vi "Koordinatenberechnung_Lichtgitter.vi"(8 "Fehler in":errorcluster, 11 "Cluster in":T1={"Initialisierung"={"Online?"=FALSE, "Grundpfad"=path "", "Kamera Oben"="", "IP-Adresse Flüssiglinse"="", "Flüssiglinse"=refnum, "Kamera Unten"="", "IP-Adresse SPS"="", "SPS-Verbindung"={"TCP Connection Ref"=refnum, "IP address"="", "timeout ms"=5000, "Connected?"=FALSE, "PLC Type"=enum."S7 1200", "Rack S7 400"=0, "Slot S7 400"=0, "PDU Size"=0, "connection semaphore"=refnum}, "IP-Adresse Lichtgitter"="", "Lichtgitter"=refnum, "Skalierungsfaktor"=0.0, "Bilder Oben"=[], "Bild Unten"=refnum, "Bild Ausschnitt Unten"=refnum}, "Einstellungen"={"Gesamtablauf gestartet"=FALSE, "i. O. Bilder speichern"=FALSE, "Bildspeicherung Offline"=FALSE, "Ausgewähltes Offline-Datum"="", "Ausgewähltes Offline-Teil"="", "Speicherpfad Bilder"=path ""}, "Artikeldaten"={"Artikelnummer"="", "Fertigungsauftrag"="", "Muster ISO"=refnum, "Belichtungszeit Referenzmarken"=0.0, "Fokus Referenzmarken"=0.0, "Belichtungszeit ISO"=0.0, "Fokus ISO"=0.0, "Belichtungszeit Unten"=0.0, "Kontaktanzahl"=0, "Aktueller Kontakt"=0, "Kontaktposition"={"x"=0.0, "y"=0.0}, "Winkel ISO"=0.0, "ISO-Muster nicht vorhanden"=FALSE}, "Werte Kamera Oben"={"Koordinatensystem"={"Punkt x-Achse"={"X"=0.0, "Y"=0.0}, "Ursprung"={"X"=0.0, "Y"=0.0}, "Punkt y-Achse"={"X"=0.0, "Y"=0.0}}, "Position Kontakt"={"x"=0.0, "y"=0.0}, "Winkel Kontakt"=0.0}, "Werte Kamera Unten"={"Prüfung Unten n. i. O."=FALSE}, "Werte Lichtgitter"={"Messwerte Referenzmarken"=[], "Mittelpunkt Referenzmarken"={"x"=0.0, "y"=0.0}, "Messwerte Kontakt"=[], "Offset"={"x"=0.0, "y"=0.0}}, "Rückmeldungen"={"Koordinaten ermittelt"=FALSE, "Vermessung Lichtgitter fertig"=FALSE, "Nachkontrolle Kamera Unten fertig"=FALSE}, "Fehler"={"Referenzen nicht gefunden"=FALSE, "Kontakt nicht gefunden"=FALSE, "Referenzen nicht in Lichtgitter"=FALSE, "Kontakt zu groß"=FALSE, "Kontakt zu klein"=FALSE}, "Statistik"={"Statistiken"=[]}, "Timer"={"Timer Start Position"=0, "Timer Start Lichtgitter"=0, "Timer Start Kamera Unten"=0}}) -> (0 "Fehler out":errorcluster, 2 "Durchmesser Kontakt (mm)":dbl format="%#.3g", 3 "Cluster out":T1={"Initialisierung"={"Online?"=FALSE, "Grundpfad"=path "", "Kamera Oben"="", "IP-Adresse Flüssiglinse"="", "Flüssiglinse"=refnum, "Kamera Unten"="", "IP-Adresse SPS"="", "SPS-Verbindung"={"TCP Connection Ref"=refnum, "IP address"="", "timeout ms"=5000, "Connected?"=FALSE, "PLC Type"=enum."S7 1200", "Rack S7 400"=0, "Slot S7 400"=0, "PDU Size"=0, "connection semaphore"=refnum}, "IP-Adresse Lichtgitter"="", "Lichtgitter"=refnum, "Skalierungsfaktor"=0.0, "Bilder Oben"=[], "Bild Unten"=refnum, "Bild Ausschnitt Unten"=refnum}, "Einstellungen"={"Gesamtablauf gestartet"=FALSE, "i. O. Bilder speichern"=FALSE, "Bildspeicherung Offline"=FALSE, "Ausgewähltes Offline-Datum"="", "Ausgewähltes Offline-Teil"="", "Speicherpfad Bilder"=path ""}, "Artikeldaten"={"Artikelnummer"="", "Fertigungsauftrag"="", "Muster ISO"=refnum, "Belichtungszeit Referenzmarken"=0.0, "Fokus Referenzmarken"=0.0, "Belichtungszeit ISO"=0.0, "Fokus ISO"=0.0, "Belichtungszeit Unten"=0.0, "Kontaktanzahl"=0, "Aktueller Kontakt"=0, "Kontaktposition"={"x"=0.0, "y"=0.0}, "Winkel ISO"=0.0, "ISO-Muster nicht vorhanden"=FALSE}, "Werte Kamera Oben"={"Koordinatensystem"={"Punkt x-Achse"={"X"=0.0, "Y"=0.0}, "Ursprung"={"X"=0.0, "Y"=0.0}, "Punkt y-Achse"={"X"=0.0, "Y"=0.0}}, "Position Kontakt"={"x"=0.0, "y"=0.0}, "Winkel Kontakt"=0.0}, "Werte Kamera Unten"={"Prüfung Unten n. i. O."=FALSE}, "Werte Lichtgitter"={"Messwerte Referenzmarken"=[], "Mittelpunkt Referenzmarken"={"x"=0.0, "y"=0.0}, "Messwerte Kontakt"=[], "Offset"={"x"=0.0, "y"=0.0}}, "Rückmeldungen"={"Koordinaten ermittelt"=FALSE, "Vermessung Lichtgitter fertig"=FALSE, "Nachkontrolle Kamera Unten fertig"=FALSE}, "Fehler"={"Referenzen nicht gefunden"=FALSE, "Kontakt nicht gefunden"=FALSE, "Referenzen nicht in Lichtgitter"=FALSE, "Kontakt zu groß"=FALSE, "Kontakt zu klein"=FALSE}, "Statistik"={"Statistiken"=[]}, "Timer"={"Timer Start Position"=0, "Timer Start Lichtgitter"=0, "Timer Start Kamera Unten"=0}})   [LabVIEW 2024]
doc: "Errechnet aus den Messwerten der Lichtgitter die aktuelle Position des Kontakts, rechnet diese dann in das Koordinatensystem der Kamera um und ermittelt den Offset, welcher von der Achse korrigiert werden muss."
uses:
  Cluster.ctl
  Kontaktmontagemodul.exe/1abvi3w/vi.lib/userDefined/High Color/IMAQdx.ctl
  Kontaktmontagemodul.exe/1abvi3w/vi.lib/DATA AHEAD/SP7/typedefs/S7 Connection.ctl
  Kontaktmontagemodul.exe/1abvi3w/vi.lib/DATA AHEAD/SP7/typedefs/PLC Type.ctl
  Kontaktmontagemodul.exe/1abvi3w/vi.lib/vision/Image Controls.llb/IMAQ Image.ctl
  Koordinatensystem.ctl
  Statistik.ctl
  Kontaktmontagemodul.exe/1abvi3w/vi.lib/Analysis/Matrix/Datatypes/RealMatrix.ctl
  Kontaktmontagemodul.exe/1abvi3w/vi.lib/Analysis/Matrix/NI_Matrix.lvlib
  Kontaktmontagemodul.exe/1abvi3w/vi.lib/DATA AHEAD/SP7/SP7.lvlib
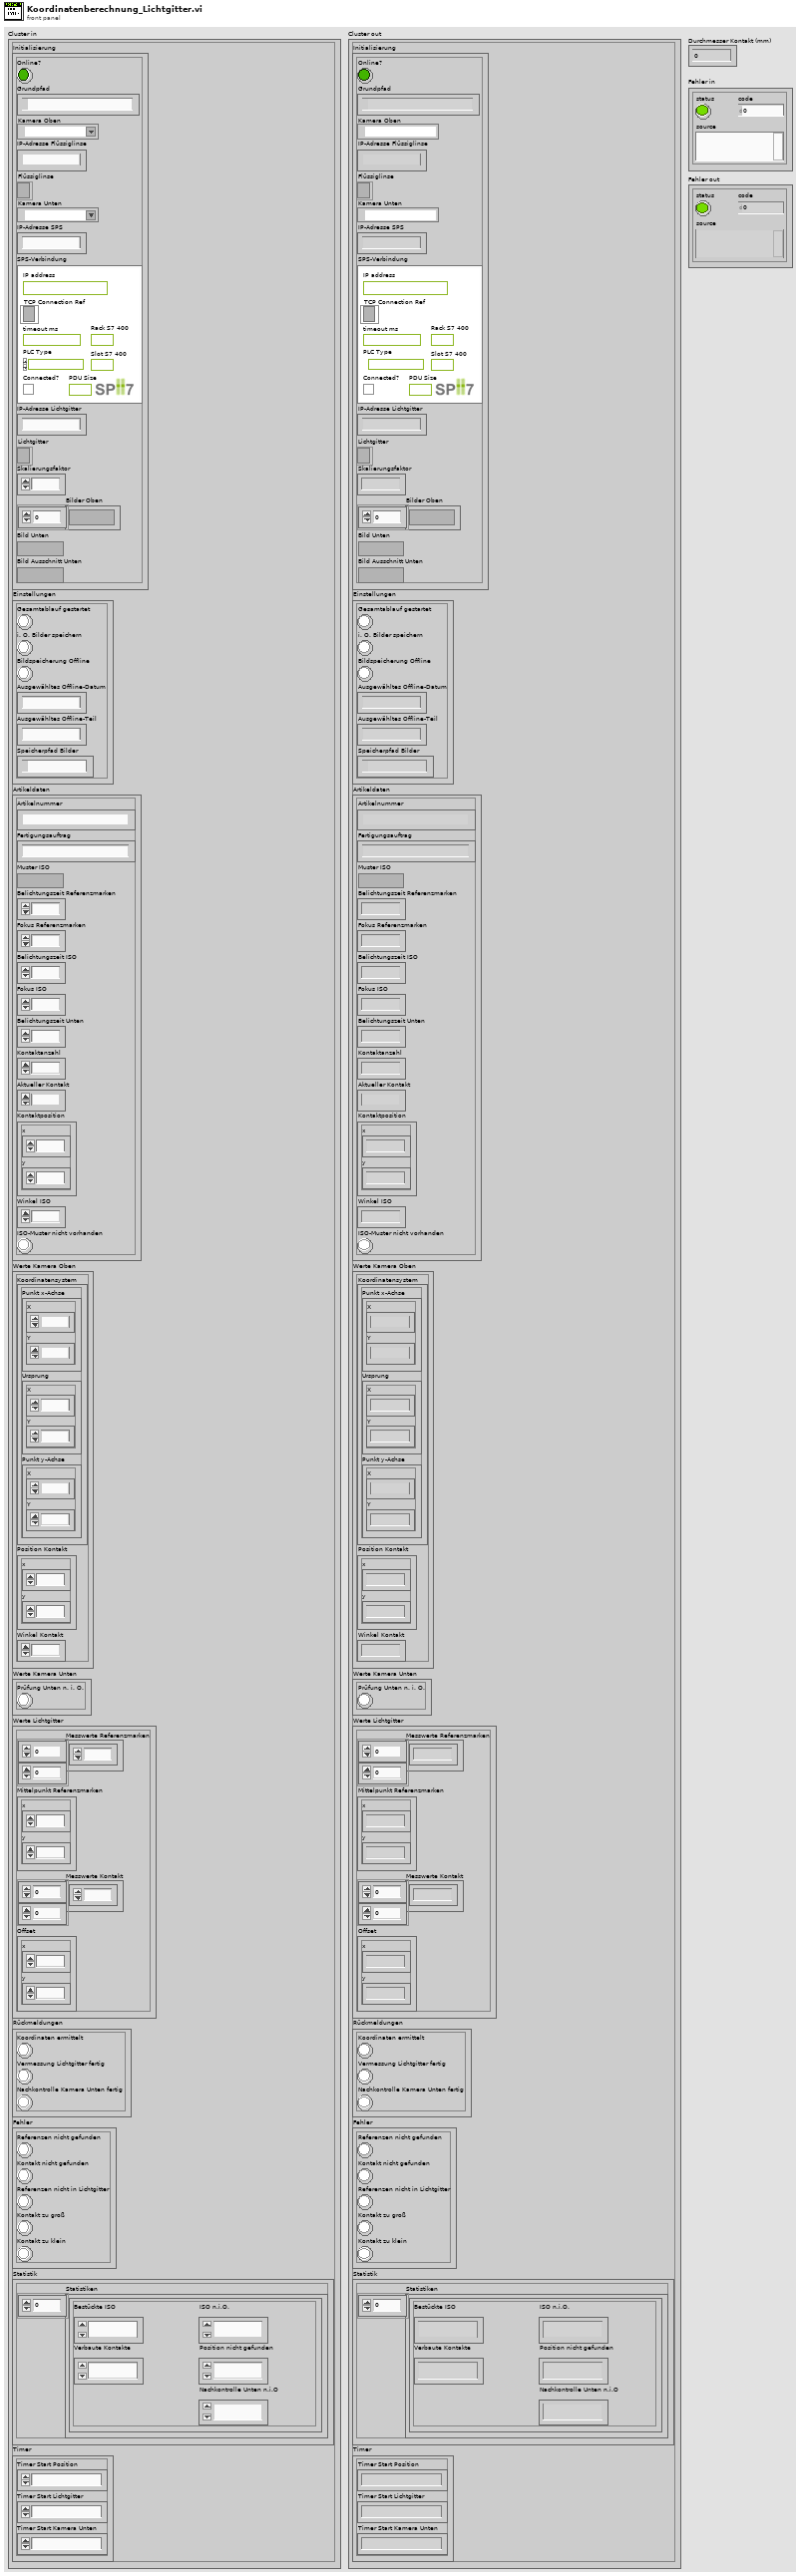
[diagram p1: front panel]
types:
  T1 = typedef "Cluster.ctl" = cluster{"Initialisierung":cluster{"Online?":bool, "Grundpfad":path, "Kamera Oben":T2, "IP-Adresse Flüssiglinse":string, "Flüssiglinse":refnum<k5>, "Kamera Unten":T2, "IP-Adresse SPS":string, "SPS-Verbindung":T3, "IP-Adresse Lichtgitter":string, "Lichtgitter":refnum<k5>, "Skalierungsfaktor":dbl, "Bilder Oben":T6[], "Bild Unten":T6, "Bild Ausschnitt Unten":T6}, "Einstellungen":cluster{"Gesamtablauf gestartet":bool, "i. O. Bilder speichern":bool, "Bildspeicherung Offline":bool, "Ausgewähltes Offline-Datum":string, "Ausgewähltes Offline-Teil":string, "Speicherpfad Bilder":path}, "Artikeldaten":cluster{"Artikelnummer":string, "Fertigungsauftrag":string, "Muster ISO":T6, "Belichtungszeit Referenzmarken":dbl, "Fokus Referenzmarken":dbl, "Belichtungszeit ISO":dbl, "Fokus ISO":dbl, "Belichtungszeit Unten":dbl, "Kontaktanzahl":u32, "Aktueller Kontakt":i16, "Kontaktposition":cluster{"x":sgl, "y":sgl}, "Winkel ISO":sgl, "ISO-Muster nicht vorhanden":bool}, "Werte Kamera Oben":cluster{"Koordinatensystem":T7, "Position Kontakt":cluster{"x":dbl, "y":dbl}, "Winkel Kontakt":dbl}, "Werte Kamera Unten":cluster{"Prüfung Unten n. i. O.":bool}, "Werte Lichtgitter":cluster{"Messwerte Referenzmarken":dbl[][], "Mittelpunkt Referenzmarken":cluster{"x":dbl, "y":dbl}, "Messwerte Kontakt":dbl[][], "Offset":cluster{"x":dbl, "y":dbl}}, "Rückmeldungen":cluster{"Koordinaten ermittelt":bool, "Vermessung Lichtgitter fertig":bool, "Nachkontrolle Kamera Unten fertig":bool}, "Fehler":cluster{"Referenzen nicht gefunden":bool, "Kontakt nicht gefunden":bool, "Referenzen nicht in Lichtgitter":bool, "Kontakt zu groß":bool, "Kontakt zu klein":bool}, "Statistik":cluster{"Statistiken":T8[]}, "Timer":cluster{"Timer Start Position":u32, "Timer Start Lichtgitter":u32, "Timer Start Kamera Unten":u32}}
  T2 = typedef "IMAQdx.ctl" = refnum<k21>
  T3 = typedef "SP7.lvlib/S7 Connection.ctl" = cluster{"TCP Connection Ref":refnum<k5>, "IP address":string, "timeout ms":i32, "Connected?":bool, "PLC Type":T4, "Rack S7 400":u8, "Slot S7 400":u8, "PDU Size":u16, "connection semaphore":T5}
  T4 = typedef "SP7.lvlib/PLC Type.ctl" = enum16{"S7 200", "S7 300/400", "S7 1200", "S7 1500", "LOGO!8"}
  T5 = typedef "Semaphore RefNum" = refnum<k1>
  T6 = typedef "IMAQ Image.ctl" = refnum<image>
  T7 = typedef "Koordinatensystem.ctl" = cluster{"Punkt x-Achse":cluster{"X":sgl, "Y":sgl}, "Ursprung":cluster{"X":sgl, "Y":sgl}, "Punkt y-Achse":cluster{"X":sgl, "Y":sgl}}
  T8 = typedef "Statistik.ctl" = cluster{"Bestückte ISO":u32, "Verbaute Kontakte":u32, "ISO n.i.O.":u32, "Nachkontrolle Unten n.i.O":u32, "Position nicht gefunden":u32}
  T9 = cluster{"Position":cluster{"X":sgl, "Y":sgl}, "Radius":dbl, "Score":dbl}
  T10 = cluster{"Farbe Kreis":u32, "Kreis ausfüllen?":bool, "Bounding Rechteck anzeigen?":bool, "Farbe Bounding Rechteck":u32}
  T11 = typedef "NI_Matrix.lvlib/RealMatrix.ctl" = dbl[][]
  T12 = cluster{"Position":cluster{"X":sgl, "Y":sgl}, "Radius":dbl, "Score":dbl}[]
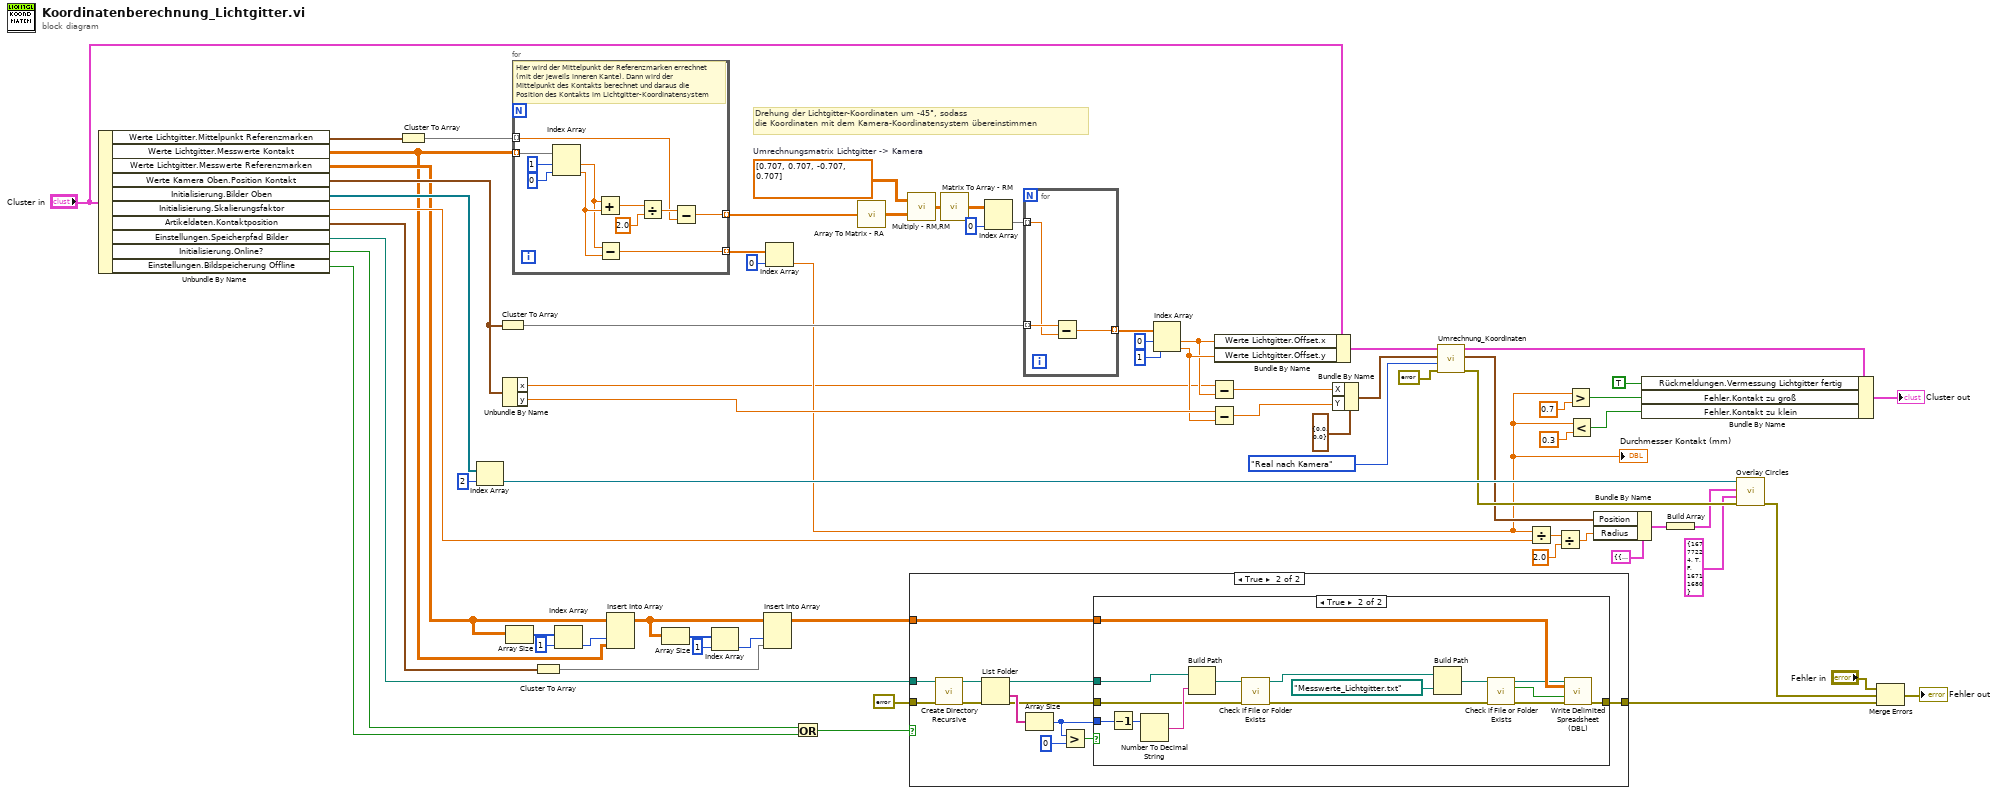
[diagram p0: block diagram]
diagram:
  w69 = T11 [[0.707, 0.707], [-0.707, 0.707]]  # Umrechnungsmatrix Lichtgitter -> Kamera
  # "Drehung der Lichtgitter-Koordinaten um -45°, sodass\ndie Koordinaten mit dem Kamera-Koordinatensystem übereinstimmen"
  n1 = Unbundle By Name("Cluster in") -> ("Werte Lichtgitter.Mittelpunkt Referenzmarken"=w10:cluster{"x":dbl, "y":dbl}, "Werte Lichtgitter.Messwerte Kontakt"=w1:dbl[][], "Werte Lichtgitter.Messwerte Referenzmarken"=w8:dbl[][], "Werte Kamera Oben.Position Kontakt"=w18:cluster{"x":dbl, "y":dbl}, "Initialisierung.Bilder Oben"=w43:T6[], "Initialisierung.Skalierungsfaktor"=w39:dbl, "Artikeldaten.Kontaktposition"=w12:cluster{"x":sgl, "y":sgl}, "Einstellungen.Speicherpfad Bilder"=w53:path, "Initialisierung.Online?"=w14:bool, "Einstellungen.Bildspeicherung Offline"=w11:bool)
  n2 = Cluster To Array(cluster=w10) -> (array=w9:dbl[])
  n3 = Index Array(array=w43, index=2) -> (element=w41:T6)
  n4 = Cluster To Array(cluster=w18) -> (array=w54:dbl[])
  n5 = Unbundle By Name(w18) -> ("x"=w19:dbl, "y"=w50:dbl)
  n6 = Array Size(array=w8) -> (size(s)=w17:i32[])
  n7 = for {
    tunnel: w1 -> [w77] mode=indexing
    tunnel: [w81] -> w70 mode=indexing
    tunnel: [w79] -> w57 mode=indexing
    tunnel: w9 -> [w72] mode=indexing
    # "Hier wird der Mittelpunkt der Referenzmarken errechnet (mit der jeweils inneren Kante). Dann wird der Mittelpunkt des Kontakts berechnet und daraus die Position des Kontakts im Lichtgitter-Koordinatensystem"
    n8 = Index Array(array=w77, index #1=1 ("index"), index #2=0 ("index")) -> (element #1=w75:dbl, element #2=w76:dbl)
    n9 = Add(x=w75, y=w76) -> (x+y=w80:dbl)
    n10 = Subtract(x=w75, y=w76) -> (x-y=w79:dbl)
    n11 = Divide(x=w80, y=2.0) -> (x/y=w78:dbl)
    n12 = Subtract(x=w78, y=w72) -> (x-y=w81:dbl)
  }
  n13 = Cluster To Array(cluster=w12) -> (array=w3:sgl[])
  n14 = Index Array(array=w17, index=1) -> (element=w15:i32)
  n15 = Insert Into Array(array=w8, index (col)=w15, new element=w1) -> (w4:dbl[][])  [unwired: 1 in]
  n16 = Array Size(array=w4) -> (size(s)=w5:i32[])
  n17 = Index Array(array=w5, index=1) -> (element=w2:i32)
  n18 = Insert Into Array(array=w4, index (col)=w2, new element=w3) -> (w7:dbl[][])  [unwired: 1 in]
  n19 = Index Array(array=w57, index=0) -> (element=w22:dbl)
  "Durchmesser Kontakt (mm)" <- w22
  n20 = Or(x=w14, y=w11) -> (x .or. y?=w13:bool)
  n21 = call "Array To Matrix - RA.vi"("Real 1D Array"=w70) -> ("Real Matrix (Column Vector)"=w68:T11)
  n22 = call "Multiply - RM,RM.vi"("Real Matrix B"=w68, "Real Matrix A"=w69) -> ("A * B"=w67:T11)
  n23 = case shown="True" w13 {
    tunnel: [w82 w94] -> w59
    tunnel: w53 -> [_ w89]
    tunnel: w7 -> [_ w87]
    tunnel: errorcluster {"status"=FALSE, "code"=0, "source"=""} ("error in") -> [w82 w86]
    frame False {
    }
    frame True {
      n24 = call "Create Directory Recursive.vi"("error in (no error)"=w86, "directory"=w89) -> ("error out"=w92:errorcluster, "directory copy"=w93:path)  [unwired: 3 in, 1 out]
      n25 = List Folder(path=w93, error in=w92) -> (path out=w91:path, folder names=w90:string[], error out=w88:errorcluster)  [unwired: 2 in, 1 out]
      n26 = Array Size(array=w90) -> (size(s)=w85:i32)
      n27 = Greater?(x=w85, y=0) -> (0:w83:bool)
      n28 = case shown="True" w83 {
        tunnel: [w95 w109] -> w94
        tunnel: w91 -> [_ w108]
        tunnel: w85 -> [_ w106]
        tunnel: w88 -> [w95 w104]
        tunnel: w87 -> [_ w101]
        frame False {
        }
        frame True {
          n29 = Decrement(x=w106) -> (x-1=w105:i32)
          n30 = Number To Decimal String(number=w105) -> (decimal integer string=w107:string)  [unwired: 1 in]
          n31 = Build Path(base path=w108, name or relative path=w107) -> (appended path=w103:path)
          n32 = call "Check if File or Folder Exists.vi"("error in (no error)"=w104, "path"=w103) -> ("error out"=w99:errorcluster, "dup path"=w102:path)  [unwired: 7 in, 1 out]
          n33 = Build Path(base path=w102, name or relative path=path "Messwerte_Lichtgitter.txt") -> (appended path=w100:path)
          n34 = call "Check if File or Folder Exists.vi"("error in (no error)"=w99, "path"=w100) -> ("error out"=w96:errorcluster, "file or folder exists?"=w98:bool, "dup path"=w97:path)  [unwired: 7 in]
          n35 = call "Write Delimited Spreadsheet (DBL).vi"("file path (dialog if empty)"=w97, "2D data"=w101, "append to file? (new file:F)"=w98, "error in (no error)"=w96) -> ("error out"=w109:errorcluster)  [unwired: 10 in, 1 out]
        }
      }
    }
  }
  n36 = call "Matrix To Array - RM.vi"("Real Matrix"=w67) -> ("Real 2D Array"=w66:dbl[][])
  n37 = Index Array(array=w66, index (col)=0 ("disabled index (col)")) -> (element=w55:dbl[])  [unwired: 1 in]
  n38 = for {
    tunnel: w55 -> [w112] mode=indexing
    tunnel: w54 -> [w113] mode=indexing
    tunnel: [w111] -> w64 mode=indexing
    n39 = Subtract(x=w113, y=w112) -> (x-y=w111:dbl)
  }
  n40 = Index Array(array=w64, index #1=0 ("index"), index #2=1 ("index")) -> (element #1=w48:dbl, element #2=w49:dbl)
  n41 = Subtract(x=w19, y=w48) -> (x-y=w46:dbl)
  n42 = Subtract(x=w50, y=w49) -> (x-y=w45:dbl)
  n43 = Bundle By Name(cluster="Cluster in", "Werte Lichtgitter.Offset.x"=w48, "Werte Lichtgitter.Offset.y"=w49) -> (w52:T1)
  n44 = Bundle By Name(cluster=cluster{"X":sgl, "Y":sgl} {"X"=0.0, "Y"=0.0} ("Koordinaten in"), "X"=w46, "Y"=w45) -> (w44:cluster{"X":sgl, "Y":sgl})
  n45 = call "Umrechnung_Koordinaten.vi"("error in"=errorcluster {"status"=FALSE, "code"=0, "source"=""}, "Richtung"=enum16{"Kamera nach Real", "Real nach Kamera"}."Real nach Kamera", "Koordinaten in"=w44, "Cluster in"=w52) -> ("error out"=w38:errorcluster, "Koordinaten out"=w34:cluster{"X":sgl, "Y":sgl}, "Cluster out"=w29:T1)  [unwired: 5 in]
  n46 = Divide(x=w22, y=w39) -> (x/y=w31:dbl)
  n47 = Divide(x=w31, y=2.0) -> (x/y=w30:dbl)
  n48 = Greater?(x=w22, y=0.7) -> (0:w24:bool)
  n49 = Less?(x=w22, y=0.3) -> (x < y?=w23:bool)
  n50 = Bundle By Name(cluster=T9 {"Position"={"X"=0.0, "Y"=0.0}, "Radius"=0.0, "Score"=0.0} ("Circle Descriptor"), "Position"=w34, "Radius"=w30) -> (w36:T9)
  n51 = Bundle By Name(cluster=w29, "Rückmeldungen.Vermessung Lichtgitter fertig"=TRUE ("Messung Lichtgitter.Vermessung Lichtgitter fertig"), "Fehler.Kontakt zu groß"=w24, "Fehler.Kontakt zu klein"=w23) -> (→"Cluster out":T1)
  n52 = Build Array(w36) -> (w35:T12)
  n53 = call "Overlay Circles.vi"("error in"=w38, "Einstellungen"=T10 {"Farbe Kreis"=16777224, "Kreis ausfüllen?"=TRUE, "Bounding Rechteck anzeigen?"=FALSE, "Farbe Bounding Rechteck"=16711680}, "Circles"=w35, "Image in"=w41) -> ("error out"=w40:errorcluster)  [unwired: 6 in, 1 out]
  n54 = Merge Errors("Fehler in", w40, w59) -> (→"Fehler out":errorcluster)
